vi "Limit Switches.vi"(9 "Motor Speed":dbl, 10 "Lower limit refnum":string="My DI RefNum", 11 "Upper limit refnum":string="My DI RefNum") -> (3 "Motor Output":dbl)   [LabVIEW 2014]
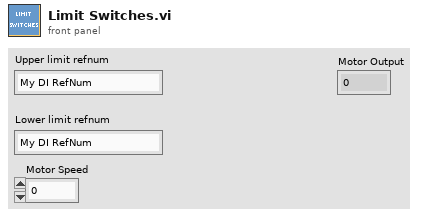
[diagram p1: front panel]
types:
  T1 = typedef "WPI_DigitalInputDevRef.ctl" = cluster{"DevStatus":errorcluster, "DIO Channel":T2, "Controller":T3}
  T2 = typedef "FPGA_DIOChannel.ctl" = enum8{"DIO 0", "DIO 1", "DIO 2", "DIO 3", "DIO 4", "DIO 5", "DIO 6", "DIO 7", "DIO 8", "DIO 9", "DIO MXP 0", "DIO MXP 1", "DIO MXP 2", "DIO MXP 3", "DIO MXP 4", "DIO MXP 5", "DIO MXP 6", "DIO MXP 7", "DIO MXP 8", "DIO MXP 9", "DIO MXP 10", "DIO MXP 11", "DIO MXP 12", "DIO MXP 13", "DIO MXP 14", "DIO MXP 15", "Invalid"}
  T3 = typedef "FPGA_TypedefDigitalModule.ctl" = enum16{"Controller 1"}
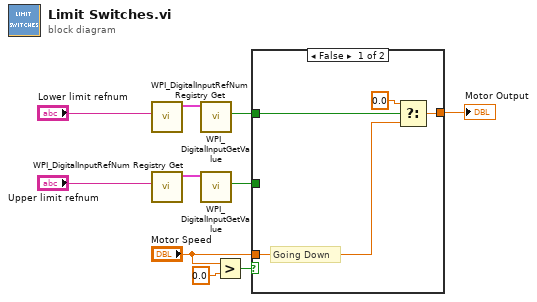
[diagram p0: block diagram]
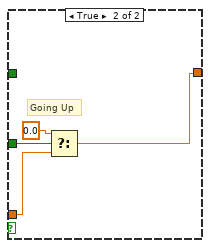
[diagram p2: hidden frame]
diagram:
  n1 = call <vilib>:"WPI_DigitalInputRefNum Registry Get.vi"("refnum name"="Lower limit refnum") -> ("DigitalInputDevRef"=w3:T1)  [unwired: 9 in, 1 out]
  n2 = call <vilib>:"WPI_DigitalInputRefNum Registry Get.vi"("refnum name"="Upper limit refnum") -> ("DigitalInputDevRef"=w10:T1)  [unwired: 9 in, 1 out]
  n3 = call <vilib>:"WPI_DigitalInputGetValue.vi"("DigitalInputDevRef"=w3) -> ("Value"=w1:bool)  [unwired: 8 in, 2 out]
  n4 = call <vilib>:"WPI_DigitalInputGetValue.vi"("DigitalInputDevRef"=w10) -> ("Value"=w2:bool)  [unwired: 8 in, 2 out]
  n5 = Greater?(x="Motor Speed", y=0.0) -> (0:w8:bool)
  n6 = case shown="False" w8 {
    tunnel: [w11 w15] -> w7
    tunnel: "Motor Speed" -> [w13 w16]
    tunnel: w2 -> [_ w18]
    tunnel: w1 -> [w12 _]
    frame False {
      # "Going Down"
      n7 = Select(t=0.0, s=w12, f=w13) -> (s? t:f=w11:dbl)
    }
    frame True {
      # "Going Up"
      n8 = Select(t=0.0, s=w18, f=w16) -> (s? t:f=w15:dbl)
    }
  }
  "Motor Output" <- w7
